vi "Assert Is Not Boolean.vi"(7 "Message (\"\")":string, 8 "error in (no error)":errorcluster, 10 "Actual":variant) -> (0 "error out":errorcluster)   [LabVIEW 2017, in "Transparent Assertions.lvlib" / "Assertions.lvlib"]
doc: "Asserts that a variable is not of Boolean type."
uses:
  Assertions.lvlib
  <vilib>/Utility/Data Type/Type Definitions/Data Type.ctl
  Constraints/LogicalNot/LogicalNot.lvclass
  Constraints/IsType/IsType.lvclass
  C:/Users/pasca/Projects/Home/TransparentAssertions/Constraint/Constraint/Constraint.lvclass
  Constraints/UnaryOperator/UnaryOperator.lvclass
  <vilib>/Utility/Data Type/NI_Data Type.lvlib
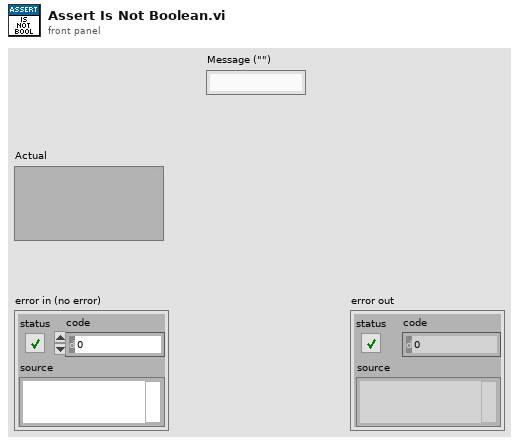
[diagram p1: front panel]
types:
  T1 = typedef "NI_Data Type.lvlib/Data Type.ctl" = enum8{"Invalid Type", "Void", "I8", "I16", "I32", "I64", "U8", "U16", "U32", "U64", "Single Float", "Double Float", "Extended Float", "Single Complex", "Double Complex", "Extended Complex", "Enum U8", "Enum U16", "Enum U32", "Enum U64", "Single Float With Unit", "Double Float With Unit", "Extended Float With Unit", "Single Complex with Unit", "Double Complex with Unit", "Extended Complex with Unit", "Boolean", "String", "Path", "Picture", "Tag", "Array", "Cluster", "Variant", "LV Variant", "Waveform", "Timestamp", "Digital Waveform", "Digital Data", "ExpressData", "Refnum", "External Data", "VI", "Poly VI", "LabVIEW Class Instance", "Fixed Point"}
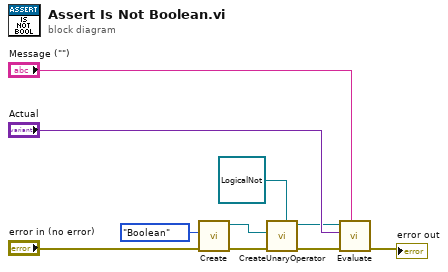
[diagram p0: block diagram]
diagram:
  n1 = call "Create.vi"("error in (no error)"="error in (no error)", "Expected"=Data_Type."Boolean") -> ("error out"=w3:errorcluster, "IsType"=w4:refnum<class "IsType.lvclass">)  [unwired: 8 in]
  n2 = call-dynamic "CreateUnaryOperator.vi"("UnaryOperator In"=refnum<class "LogicalNot.lvclass"> refnum, "error in (no error)"=w3, "Constraint"=w4) -> ("error out"=w2:errorcluster, "UnaryOperator"=w1:refnum<class "UnaryOperator.lvclass">)  [unwired: 7 in]
  n3 = call-dynamic "Evaluate.vi"("Message (\"\")"="Message (\"\")", "error in (no error)"=w2, "Actual"="Actual", "Constraint in"=w1) -> ("error out"=→"error out":errorcluster)  [unwired: 6 in, 1 out]
